vi "FTW-MessagePayload-Deserialize.vi"(0 "Serialized Message String":string, 11 "error in":errorcluster) -> (4 "Message":T1, 15 "error out":errorcluster)   [LabVIEW 2013]
uses:
  FTW-MessagePayload.ctl
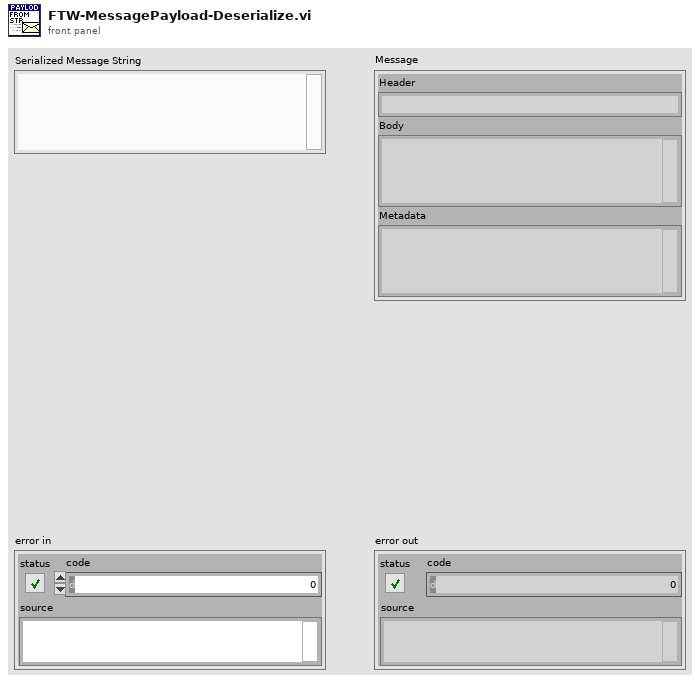
[diagram p1: front panel]
types:
  T1 = typedef "FTW-MessagePayload.ctl" = cluster{"Header":string, "Body":string, "Metadata":string}
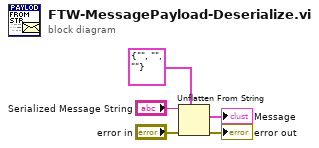
[diagram p0: block diagram]
diagram:
  n1 = Unflatten From String(type=T1 {"Header"="", "Body"="", "Metadata"=""} ("Message"), binary string="Serialized Message String", error in (no error)="error in") -> (value=→"Message":T1, error out=→"error out":errorcluster)  [unwired: 2 in, 1 out]
